vi "Set Server Certificate File.vi"(10 "Server Certificate File (.crt)":path, 11 "OOP Server in":refnum<class "server12.lvclass">) -> (3 "OOP Server out":refnum<class "server12.lvclass">)   [LabVIEW 2020, in "server12.lvlib" / "server12.lvclass"]
uses:
  server12.lvclass
  server12.lvclass/server12.ctl
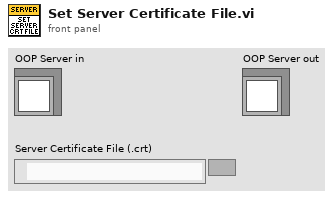
[diagram p1: front panel]
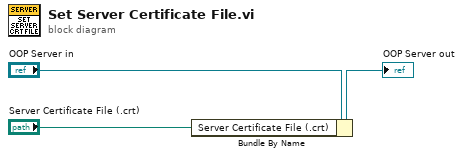
[diagram p0: block diagram]
diagram:
  n1 = Bundle By Name(cluster="OOP Server in", "Server Certificate File (.crt)"="Server Certificate File (.crt)") -> (→"OOP Server out":refnum<class "server12.lvclass">)
